vi "Save EEPROM To File.vi"(11 "cFileName":string) -> (2 "function return":u32, 3 "cFileName out":string)   [LabVIEW 2018, in "AndorSDK.lvlib"]
doc: "EXPNETTYPE unsigned int WINAPI SaveEEPROMToFile(char * cFileName);"
uses:
  AndorSDK.lvlib
  ATMCD32D.dll
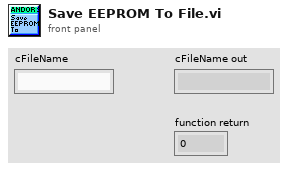
[diagram p1: front panel]
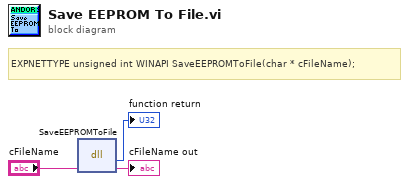
[diagram p0: block diagram]
diagram:
  # "EXPNETTYPE unsigned int WINAPI SaveEEPROMToFile(char * cFileName);"
  n1 = dll-call lib="PTH2babs E\nPersönliches02 - Arbeit03-HiwijobsLabviewCodelibANDOR\tAndor SDK\nATMCD32D.*" fn="SaveEEPROMToFile"("cFileName"="cFileName") -> (→"function return":u32, "cFileName"=→"cFileName out":string)  [unwired: 3 in, 2 out]
